vi "Emergency kill loop by reference.vi"(9 "Quit early notifier":refnum<notifier>, 11 "VI reference in":refnum<vi>) -> (0 "error out":errorcluster)   [LabVIEW 2018]
doc: "This VI is reentrant so it can be present on multiple VIs with visible front panels at the same time and not have issues. It waits for the VI whose reference is passed in to see if Control-Shift-K is pressed. If so, gives an option to hard-stop the entire software execution.\n\nOptionally, you can create a Boolean Notifier reference and pass that into this VI. If the reference is functional and the value is True, then this VI exits within 100 ms. This input should be used on any panel containing this VI that may need to close prior to the entire program stopping at once.\n\nOtherwise, waits for the shutdown event and quits.\n\nNote: This VI includes an error output for dataflow purposes only, and never outputs an actual error. It does not have an error input because it is designed to always run, and run immediately."
uses:
  References/Fiber Auto Collimation References.lvclass
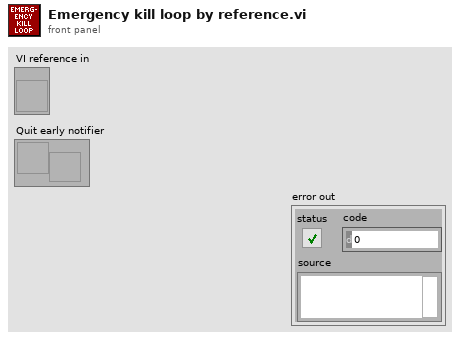
[diagram p1: front panel]
types:
  T1 = cluster{"Shift":bool, "Ctrl":bool, "Alt":bool, "Cmd":bool, "Opt":bool}
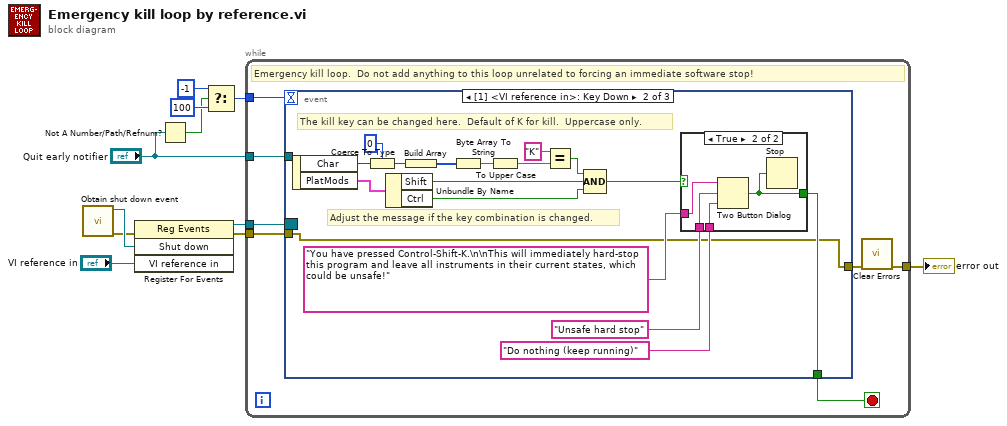
[diagram p0: block diagram]
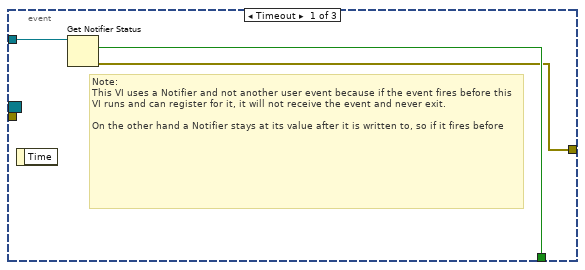
[diagram p2: hidden frame]
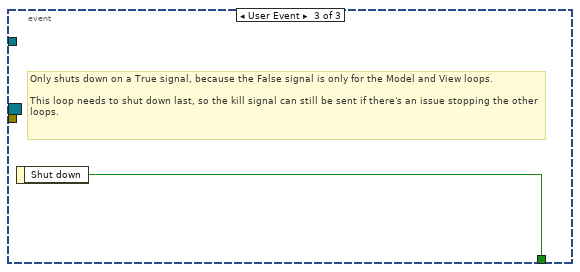
[diagram p4: hidden frame]
diagram:
  n1 = call "Obtain shut down event.vi"() -> ("error out"=w8:errorcluster, "Shut down"=w9:refnum<user-event>)  [unwired: 10 in]
  n2 = register-events(error in=w8, w9, "VI reference in") -> (reference out=w10:refnum<event-registration>, error out=w1:errorcluster)  [unwired: 1 in]
  n3 = Not A Number/Path/Refnum?(number/path/refnum="Quit early notifier") -> (NaN/Path/Refnum?=w4:bool)
  n4 = Select(t=-1, s=w4, f=100) -> (s? t:f=w5:i32)
  n5 = while {
    tunnel: [w17] -> w7
    tunnel: w10 -> [w16]
    tunnel: w5 -> [w15]
    tunnel: "Quit early notifier" -> [w14]
    tunnel: w1 -> [w12]
    stop <- w18 stop-if-true
    # "Emergency kill loop.  Do not add anything to this loop unrelated to forcing an immediate software stop!"
    n6 = event "Kill" shown="[1] <VI reference in>: Key Down" {
      selector: w16 -> [_ _ _]
      dyn-events: _ -> [_ _ _]
      timeout: w15 -> [_ _ _]
      tunnel: [w20 w26 w43] -> w18
      tunnel: w14 -> [w21 _ _]
      tunnel: [w19 w22 _] -> w13
      tunnel: w12 -> [_ w22 _]
      event Timeout {
        # "Note:\nThis VI uses a Notifier and not another user event because if the event fires before this VI runs and can register for it, it will not receive the event and never exit.\n\nOn the other hand a Notifier stays at its value after it is written to, so if it fires before"
        n7 = event-data() -> ()  [unwired: 1 in, 1 out]
        n8 = Get Notifier Status(notifier=w21) -> (current notification=w20:bool, error out=w19:errorcluster)  [unwired: 1 in, 3 out]
      }
      event Key Down {
        # "Adjust the message if the key combination is changed."
        # "The kill key can be changed here.  Default of K for kill.  Uppercase only."
        n9 = event-data() -> ("Char"=w38:i16, "PlatMods"=w31:T1)  [unwired: 1 in]
        n10 = Coerce To Type(0:w38, 1:u8 0) -> (2:w37:u8)
        n11 = Unbundle By Name(w31) -> ("Shift"=w29:bool, "Ctrl"=w28:bool)
        n12 = Build Array(w37) -> (w35:u8[])
        n13 = Byte Array To String(unsigned byte array=w35) -> (string=w34:string)
        n14 = To Upper Case(1:w34) -> (0:w33:string)
        n15 = Equal?(x="K", y=w33) -> (x = y?=w30:bool)
        n16 = Compound Arithmetic op=AND(w30, w29, w28) -> (w27:bool)
        n17 = case shown="True" w27 {
          tunnel: [_ w42] -> w26
          tunnel: "You have pressed Control-Shift-K.\n\nThis will immediately hard-stop this program and leave all instruments in their current states, which could be unsafe!" ("message") -> [_ w41]
          tunnel: "Unsafe hard stop" -> [_ w40]
          tunnel: "Do nothing (keep running)" -> [_ w39]
          frame False {
          }
          frame True {
            n18 = Two Button Dialog(message=w41, 1:w39, 2:w40) -> (T button?=w42:bool)
            n19 = Stop(stop? (T)=w42) -> ()
          }
        }
      }
      event User Event {
        # "Only shuts down on a True signal, because the False signal is only for the Model and View loops.\n\nThis loop needs to shut down last, so the kill signal can still be sent if there's an issue stopping the other loops."
        n20 = event-data() -> ("Shut down"=w43:bool)  [unwired: 1 in]
      }
    }
    n21 = call <vilib>:"Clear Errors.vi"("error in (no error)"=w13) -> ("error out"=w17:errorcluster)  [unwired: 5 in, 1 out]
  }
  "error out" <- w7
